vi "Add to Constants Base basic.vi"(8 "error in (no error)":errorcluster, 9 "Value":dbl, 10 "Constant Name":string, 11 "Constants Map":T1) -> (0 "Error out":errorcluster, 3 "Constants Map out":T1)   [LabVIEW 2013]
uses:
  Constants Map typedef.ctl
  Constants typedef V2.ctl
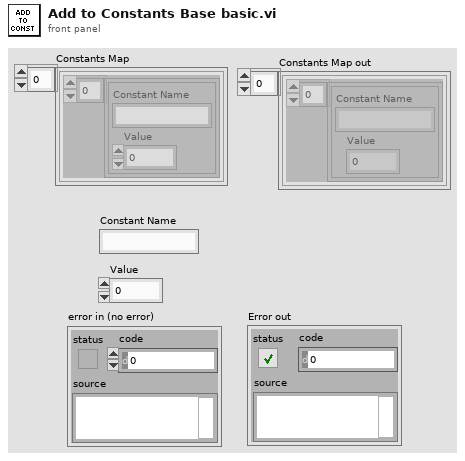
[diagram p1: front panel]
types:
  T1 = typedef "Constants Map typedef.ctl" = cluster{T2[]}[]
  T2 = typedef "Constants typedef V2.ctl" = cluster{"Constant Name":string, "Value":dbl}
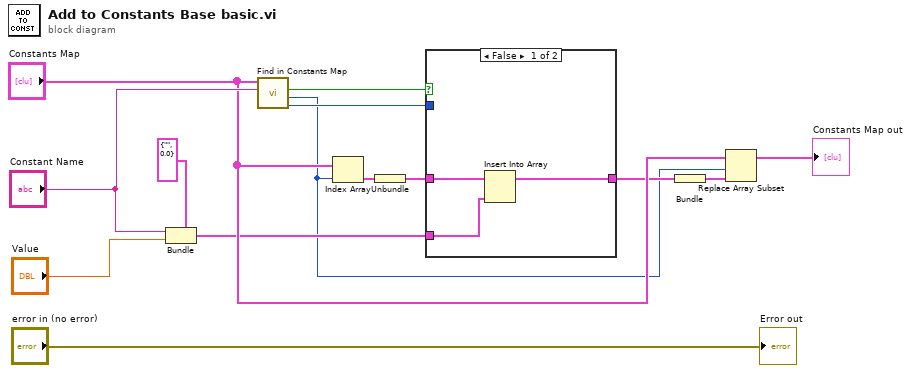
[diagram p0: block diagram]
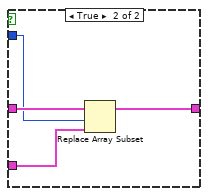
[diagram p2: hidden frame]
diagram:
  n1 = Bundle(cluster=T2 {"Constant Name"="", "Value"=0.0} ("Constants"), "Constant Name"="Constant Name", "Value"="Value") -> (w6:T2)
  n2 = call "Find in Constants Map.vi"("Constant Name"="Constant Name", "Constants Map"="Constants Map") -> ("index"=w5:i32, "Hash Index"=w2:i32, "Did it find it"=w10:bool)  [unwired: 6 in, 1 out]
  n3 = Index Array(array="Constants Map", index=w2) -> (element=w8:cluster{T2[]})
  n4 = Unbundle(w8) -> (w7:T2[])
  n5 = case shown="False" w10 {
    tunnel: w7 -> [w17 w21]
    tunnel: w6 -> [w16 w20]
    tunnel: w5 -> [_ w19]
    tunnel: [w15 w18] -> w4
    frame False {
      n6 = Insert Into Array(array=w17, new element=w16) -> (w15:T2[])  [unwired: 1 in]
    }
    frame True {
      n7 = Replace Array Subset(array=w21, new element=w20, index=w19) -> (w18:T2[])
    }
  }
  n8 = Bundle(w4) -> (w3:cluster{T2[]})  [unwired: 1 in]
  n9 = Replace Array Subset(array="Constants Map", new element=w3, index=w2) -> (→"Constants Map out":T1)
  "Error out" <- "error in (no error)"
